vi "XPARTD_XPARTDServer.vi"(5 "timeout":i32=5000, 7 "error in (no error)":errorcluster, 9 "cmd":string) -> (0 "error out":errorcluster, 2 "response":string)   [LabVIEW 2016]
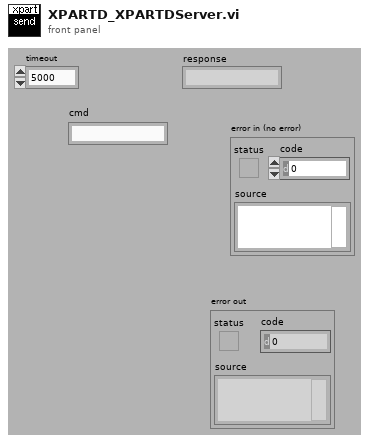
[diagram p1: front panel]
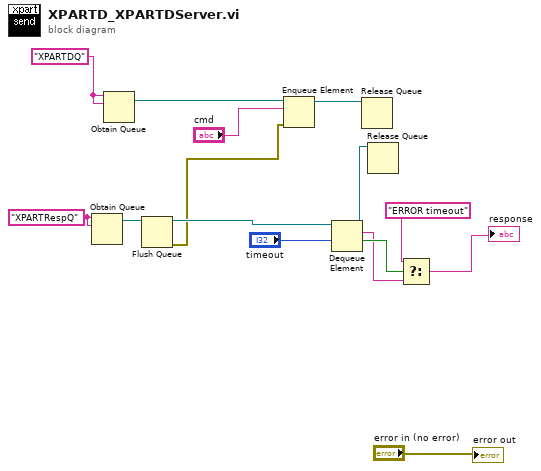
[diagram p0: block diagram]
diagram:
  w13 = "XPARTRespQ" ("name (unnamed)")
  w14 = "XPARTDQ" ("name (unnamed)")
  n1 = Obtain Queue(name (unnamed)=w13, element data type=w13) -> (queue out=w11:refnum<queue>)  [unwired: 3 in, 2 out]
  n2 = Obtain Queue(name (unnamed)=w14, element data type=w14) -> (queue out=w12:refnum<queue>)  [unwired: 3 in, 2 out]
  n3 = Flush Queue(queue=w11) -> (queue out=w10:refnum<queue>, error out=w8:errorcluster)  [unwired: 1 in, 1 out]
  n4 = Enqueue Element(queue=w12, element="cmd", error in (no error)=w8) -> (queue out=w2:refnum<queue>)  [unwired: 3 out]
  n5 = Dequeue Element(queue=w10, timeout in ms (-1)="timeout") -> (queue out=w1:refnum<queue>, element=w5:string, timed out?=w6:bool)  [unwired: 1 in, 1 out]
  n6 = Release Queue(queue=w2) -> ()  [unwired: 1 in, 4 out]
  n7 = Release Queue(queue=w1) -> ()  [unwired: 1 in, 4 out]
  n8 = Select(t="ERROR timeout", s=w6, f=w5) -> (s? t:f=→"response":string)
  "error out" <- "error in (no error)"
